vi "File_setup.vi"(4 "Measurement is top level?":bool, 5 "Results file":path, 6 "Raw data file":path, 7 "setup":T1, 8 "File":T3) -> (0 "Results file output":path, 1 "Raw data file output":path, 2 "Raw data option":enum16{"Save raw data", "Raw data not saved"}(ring), 3 "File output":T2(ring))   [LabVIEW 2010]
uses:
  Controls/Save_Data.ctl
  Controls/Setup.ctl
  Controls/Post_Process.ctl
  Globals/Meas_global.vi
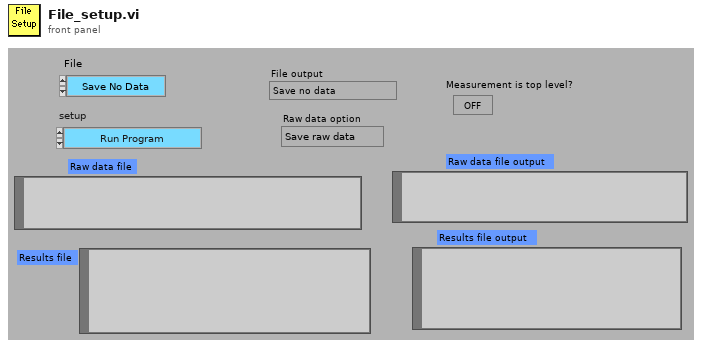
[diagram p1: front panel]
types:
  T1 = typedef "Setup.ctl" = enum16{"Run Program", "Show Setup", "Save Current Setup", "Setup Front Panel"}
  T2 = enum16{"Save no data", "Save data in new files", "Save data in existing files"}
  T3 = typedef "Save_Data.ctl" = enum16{"Save No Data", "Save Data"}
  T4 = typedef "Post_Process.ctl" = enum16{"Take New Data", "Post Process Raw Data File"}
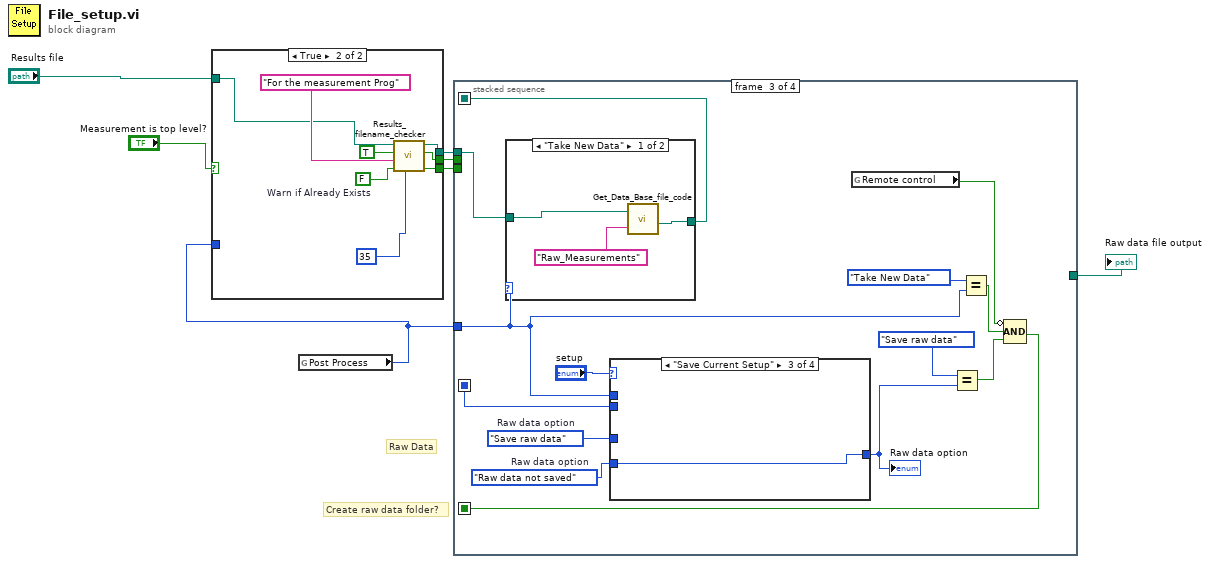
[diagram p0: block diagram]
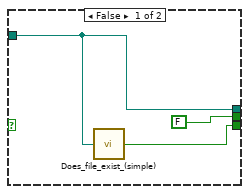
[diagram p2: hidden frame]
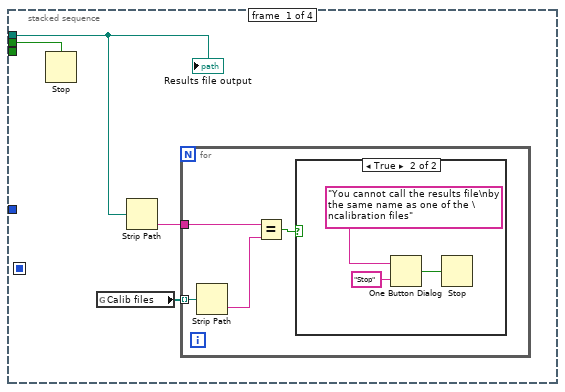
[diagram p3: hidden frame]
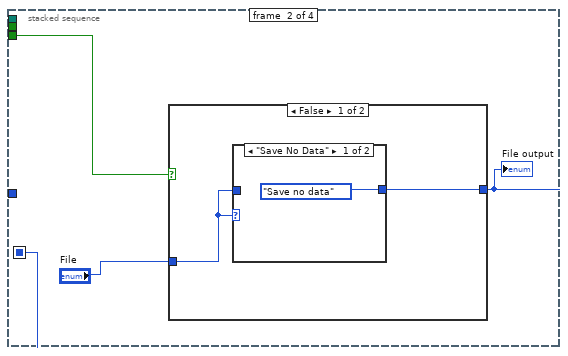
[diagram p5: hidden frame]
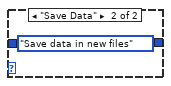
[diagram p6: hidden frame]
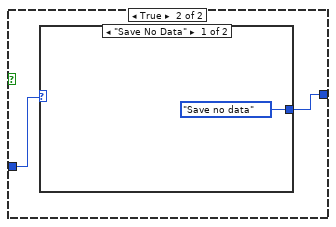
[diagram p7: hidden frame]
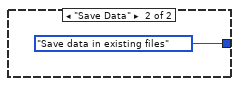
[diagram p8: hidden frame]
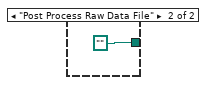
[diagram p9: hidden frame]
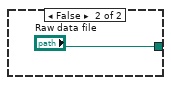
[diagram p17: hidden frame]
diagram:
  # "Create raw data folder?"
  # "Raw Data"
  n1 = global read "Meas_global.vi" "Post Process"() -> (w3:T4)
  n2 = case shown="True" "Measurement is top level?" {
    tunnel: [w10 w18] -> w7
    tunnel: [w9 w17] -> w6
    tunnel: [FALSE ("cancelled") w16] -> w4
    tunnel: w3 -> [_ _]
    tunnel: "Results file" -> [w10 w11]
    frame False {
      n3 = call "Does_file_exist_(simple).vi"("Pathname"=w10) -> ("exists?"=w9:bool)
    }
    frame True {
      w13 = FALSE  # Warn if Already Exists
      n4 = call "Results_filename_checker.vi"("Filelength"=35, "Warn if Already Exists"=w13, "Comment"="For the measurement Prog", "Show Error handler"=TRUE, "Results file"=w11) -> ("exists?"=w17:bool, "cancelled"=w16:bool, "Results file output"=w18:path)  [unwired: 1 out]
    }
  }
  n5 = stacked-sequence {
    seq-local: [_ w31 _ _] -> [_ _ w54 _]
    seq-local: [_ _ w45 _] -> [_ _ _ w77]
    seq-local: [_ _ w41 _] -> [_ _ _ w75]
    tunnel: w3 -> [_ _ w42 _]
    tunnel: w7 -> [w21 _ w44 w78]
    tunnel: w6 -> [_ w30 _ _]
    tunnel: [_ _ _ w76] -> w5
    tunnel: w4 -> [w19 _ _ _]
    frame #0 {
      n6 = Stop(stop? (T)=w19) -> ()
      n7 = global read "Meas_global.vi" "Calib files"() -> (w22:path[])
      n8 = Strip Path(path=w21) -> (name=w20:string)  [unwired: 1 out]
      n9 = for {
        tunnel: w22 -> [w24] mode=indexing
        tunnel: w20 -> [w26]
        n10 = Strip Path(path=w24) -> (name=w23:string)  [unwired: 1 out]
        n11 = Equal?(x=w26, y=w23) -> (x = y?=w25:bool)
        n12 = case shown="True" w25 {
          frame False {
          }
          frame True {
            n13 = One Button Dialog(message="You cannot call the results file\nby the same name as one of the \ncalibration files", button name ("OK")="Stop") -> (true=w27:bool)
            n14 = Stop(stop? (T)=w27) -> ()
          }
        }
      }
      "Results file output" <- w21
    }
    frame #1 {
      n15 = case shown="False" w30 {
        tunnel: "File" -> [w33 w38]
        tunnel: [w34 w37] -> w31
        frame False {
          n16 = case shown="\"Save No Data\"" w33 {
            tunnel: [T2."Save no data" ("File output") T2."Save data in new files" ("File output")] -> w34
            tunnel: w33 -> [_ _]
            frame "Save No Data" {
            }
            frame "Save Data" {
            }
          }
        }
        frame True {
          n17 = case shown="\"Save No Data\"" w38 {
            tunnel: [T2."Save no data" ("File output") T2."Save data in existing files" ("File output")] -> w37
            frame "Save No Data" {
            }
            frame "Save Data" {
            }
          }
        }
      }
      "File output" <- w31
    }
    frame #2 {
      w52 = enum16{"Save raw data", "Raw data not saved"}."Raw data not saved"  # Raw data option
      w53 = enum16{"Save raw data", "Raw data not saved"}."Save raw data"  # Raw data option
      n18 = case shown="\"Take New Data\"" w42 {
        tunnel: w44 -> [w57 _]
        tunnel: [w56 path ""] -> w41
        frame "Take New Data" {
          n19 = call "Get_Data_Base_file_code.vi"("Results Filename"=w57, "Data Type"="Raw_Measurements") -> ("Raw Data File Name"=w56:path)  [unwired: 3 out]
        }
        frame "Post Process Raw Data File" {
        }
      }
      n20 = case shown="\"Save Current Setup\"" "setup" {
        tunnel: [w63 w72 w73 w74] -> w50
        tunnel: w52 -> [w62 w72 w73 w74]
        tunnel: w53 -> [w61 _ _ _]
        tunnel: w42 -> [w60 _ _ _]
        tunnel: w54 -> [w59 _ _ _]
        frame "Run Program" {
          n21 = case shown="\"Take New Data\"" w60 {
            tunnel: w59 -> [w67 _]
            tunnel: [w66 w71] -> w63
            tunnel: w61 -> [w65 _]
            tunnel: w62 -> [w64 w71]
            frame "Take New Data" {
              n22 = case shown="\"Save no data\"" w67 {
                tunnel: [w68 w69 w70] -> w66
                tunnel: w64 -> [w68 _ _]
                tunnel: w65 -> [_ w69 w70]
                frame "Save no data" {
                }
                frame "Save data in new files" {
                }
                frame "Save data in existing files" {
                }
              }
            }
            frame "Post Process Raw Data File" {
            }
          }
        }
        frame "Show Setup" {
        }
        frame "Save Current Setup" {
        }
        frame "Setup Front Panel" {
        }
      }
      "Raw data option" <- w50
      n23 = global read "Meas_global.vi" "Remote control"() -> (w43:bool)
      n24 = Equal?(x=enum16{"Save raw data", "Raw data not saved"}."Save raw data" ("Raw data option"), y=w50) -> (x = y?=w47:bool)
      n25 = Equal?(x=Post_Process."Take New Data" ("Post Process"), y=w42) -> (x = y?=w46:bool)
      n26 = Compound Arithmetic op=AND(invert w43, w46, w47) -> (w45:bool)
    }
    frame #3 {
      n27 = case shown="True" w77 {
        tunnel: [w79 "Raw data file"] -> w76
        tunnel: w78 -> [_ _]
        tunnel: w75 -> [w79 _]
        frame True {
        }
        frame False {
        }
      }
    }
  }
  "Raw data file output" <- w5
